vi "wireErrorTerminalsInEmptyCase.vi"(8 "error in (no error)":errorcluster, 10 "reference out_CDSNew":refnum<vi>, 11 "VI in":refnum<class "VI.lvclass">) -> (0 "error out":errorcluster, 3 "VI out":refnum<class "VI.lvclass">)   [LabVIEW 2016, in "VI.lvclass"]
uses:
  VI.lvclass
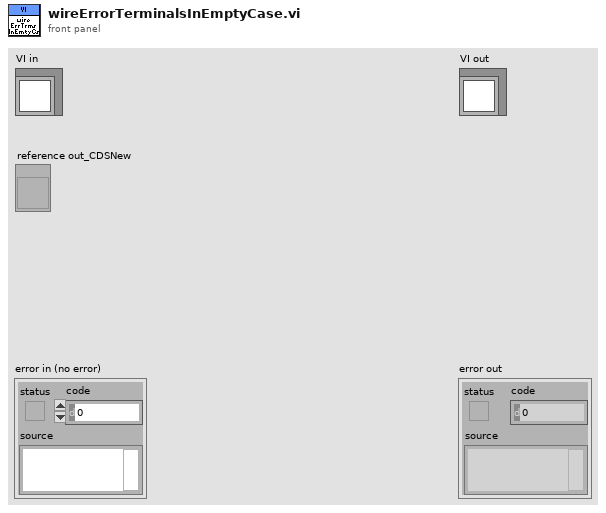
[diagram p1: front panel]
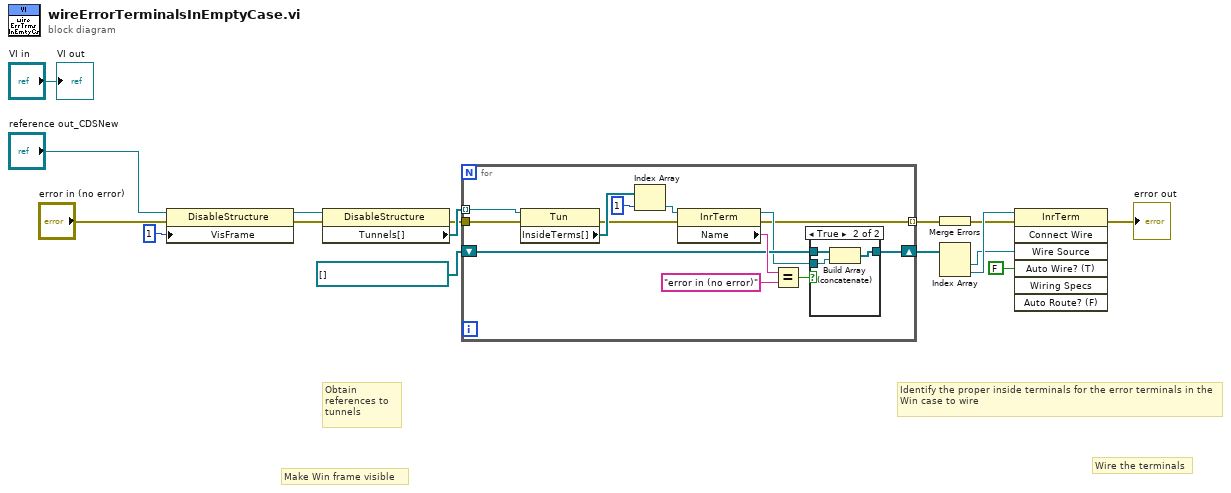
[diagram p0: block diagram]
diagram:
  # "Wire the terminals"
  # "Identify the proper inside terminals for the error terminals in the Win case to wire"
  # "Obtain references to tunnels"
  # "Make Win frame visible"
  n1 = property class="DisableStructure"(reference="reference out_CDSNew", error in="error in (no error)", "VisFrame"=i16 1 ("Active Frame")) -> (reference out=w14:refnum<vi>, error out=w7:errorcluster)
  n2 = property class="DisableStructure"(reference=w14, error in=w7) -> (error out=w6:errorcluster, "Tunnels[]"=w13:refnum<vi>[])  [unwired: 1 out]
  n3 = for {
    tunnel: w13 -> [w29] mode=indexing
    shift-right: [w21] -> w11
    shift-left: refnum<vi>[] [] ("Array 6") -> [w23]
    tunnel: w6 -> [w19]
    tunnel: [w17] -> w5 mode=indexing
    n4 = property class="Tun"(reference=w29, error in=w19) -> (error out=w18:errorcluster, "InsideTerms[]"=w28:refnum<vi>[])  [unwired: 1 out]
    n5 = Index Array(array=w28, index=1) -> (element=w26:refnum<vi>)
    n6 = property class="InrTerm"(reference=w26, error in=w18) -> (reference out=w20:refnum<vi>, error out=w17:errorcluster, "Name"=w25:string)
    n7 = Equal?(x=w25, y="error in (no error)") -> (x = y?=w22:bool)
    n8 = case shown="True" w22 {
      tunnel: w23 -> [w30 w33]
      tunnel: [w30 w32] -> w21
      tunnel: w20 -> [_ w31]
      frame False {
      }
      frame True {
        n9 = Build Array (concatenate)(w33, w31) -> (w32:refnum<vi>[])
      }
    }
  }
  n10 = Merge Errors(w5) -> (w4:errorcluster)
  n11 = Index Array(array=w11) -> (element #1=w9:refnum<vi>, element #2=w10:refnum<vi>)  [unwired: 2 in]
  n12 = invoke class="InrTerm" method="Connect Wire"(reference=w10, error in=w4, "Wire Source"=w9, "Auto Wire? (T)"=FALSE) -> (error out=→"error out":errorcluster)  [unwired: 3 in, 6 out]
  "VI out" <- "VI in"
